vi "read_compare.vi"(3 "统一指令集":T1, 6 "指令":string, 7 "应答":string, 8 "baud rate (9600)":u32=9600 caption="波特率(9600)", 9 "parity (0:none)":enum16{"None", "Odd", "Even", "Mark", "Space"}(ring) caption="奇偶（0:无）", 10 "stop bits (10: 1 bit)":u16(ring)=10 caption="停止位（10: 1位）" items=["1.0"=10, "1.5"=15, "2.0"=20], 11 "VISA resource name":refnum<visa-resource-name> caption="VISA资源名称") -> (1 "码词":string, 2 "error out":errorcluster, 4 "布尔":bool, 5 "VISA resource name out":refnum<visa-resource-name>)   [LabVIEW 2020]
uses:
  <vilib>/Instr/_visa.llb/VISA Set IO Buffer Mask.ctl
  <vilib>/Instr/_visa.llb/VISA Configure Serial Port (Instr).vi
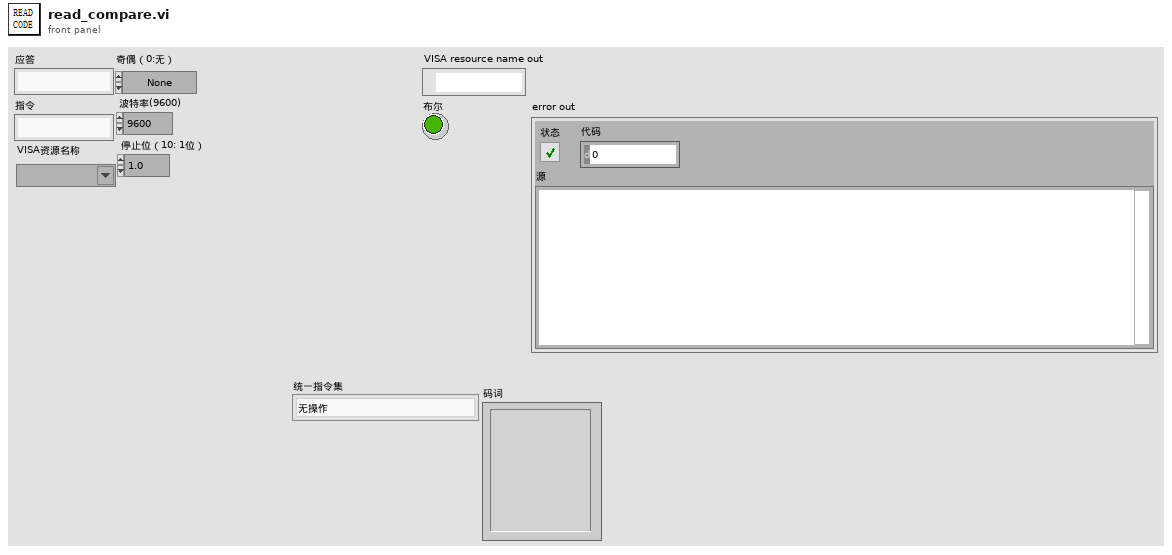
[diagram p1: front panel]
types:
  T1 = typedef "统一指令集.ctl" = enum16{"无操作", "自定义", "波特率切换为9600", "波特率切换为115200", "拍图/解码", "取图", "电平触发模式", "连续读码模式", "睡眠模式", "获取图像分辨率", "开启RTS与CTS流控", "无流控", "感应模式", "红外感应模式", "图像感应模式", "图像与红外感应模式", "切换为串口", "切换为CDC", "关闭照明灯", "开启照明灯", "照明灯常亮", "关闭瞄准灯", "开启瞄准灯", "开启设置码", "连续读码模式2", "触发模式", "0390命令识读模式", "0390连续识读模式", "查询产品序列号", "查询SN空间大小", "产品信息修改开关", "设置产品序列号", "删除序列号", "0390单芯片开启EEPROM写入", "0390单芯片关闭EEPROM写入", "0390单芯片写入产品序列号", "0390单芯片查询产品序列号"}
  T2 = typedef "VISA Set IO Buffer Mask.ctl" = u16
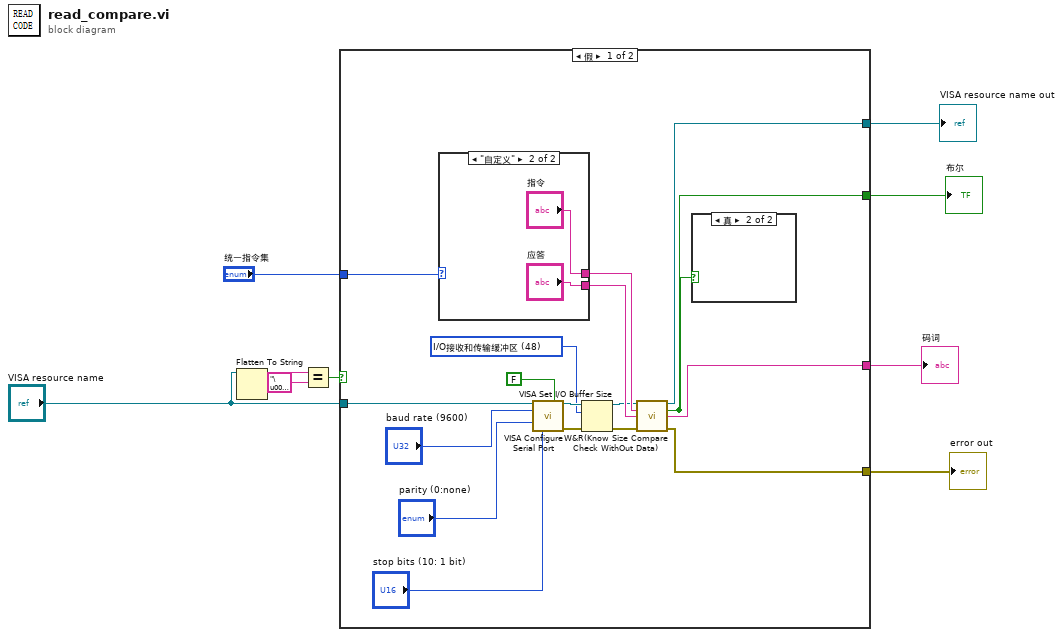
[diagram p0: block diagram]
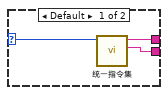
[diagram p2: hidden frame]
diagram:
  n1 = Flatten To String(anything="VISA resource name") -> (data string=w9:string)  [unwired: 3 in, 2 out]
  n2 = Equal?(x=w9, y="\u0000\u0000\u0000\u0000") -> (x = y?=w8:bool)
  n3 = case shown="假" w8 {
    tunnel: "VISA resource name" -> [w16 _]
    tunnel: [w14 _] -> w6
    tunnel: [w13 _] -> w5
    tunnel: [w12 _] -> w4
    tunnel: [w11 _] -> w3
    tunnel: "统一指令集" -> [w10 _]
    frame False {
      w17 = T2 48 items=["I/O接收缓冲区"=16, "I/O传输缓冲区"=32, "I/O接收和传输缓冲区"=48] ("Mask")
      n4 = case shown="\"自定义\"" w10 {
        selector: w10 -> [w29 _]
        tunnel: [w28 "指令"] -> w21
        tunnel: [w27 "应答"] -> w22
        frame Default {
          n5 = call "统一指令集.vi"("统一指令集"=w29) -> ("应答"=w27:string, "指令"=w28:string)  [unwired: 8 in, 1 out]
        }
        frame "自定义" {
        }
      }
      n6 = call-poly "VISA Configure Serial Port"("VISA resource name"=w16, "Enable Termination\nChar (T)"=FALSE ("Enable Termination\nChar (T)"), "baud rate (9600)"="baud rate (9600)", "parity (0:none)"="parity (0:none)", "stop bits (10: 1 bit)"="stop bits (10: 1 bit)") -> ("VISA resource name out"=w18:refnum<visa-resource-name>, "error out"=w19:errorcluster)  [unwired: 9 in]
      n7 = VISA Set I/O Buffer Size(VISA resource name=w18, mask (16)=w17, error in (no error)=w19) -> (VISA resource name out=w20:refnum<visa-resource-name>, error out=w23:errorcluster)  [unwired: 1 in]
      n8 = call "W&R(Know Size Compare Check WithOut Data).vi"("VISA resource name in"=w20, "写入指令/数据"=w21, "比较校验"=w22, "error in"=w23) -> ("VISA resource name out"=w13:refnum<visa-resource-name>, "布尔"=w14:bool, "码词"=w12:string, "error out"=w11:errorcluster)  [unwired: 8 in]
      n9 = case shown="真" w14 {
        frame False {
        }
        frame True {
        }
      }
    }
    frame True {
    }
  }
  "布尔" <- w6
  "VISA resource name out" <- w5
  "码词" <- w4
  "error out" <- w3
